vi "random_number.vi"() -> ()   [LabVIEW 2018]
panel:
  out "波形图":dbl[](graph)
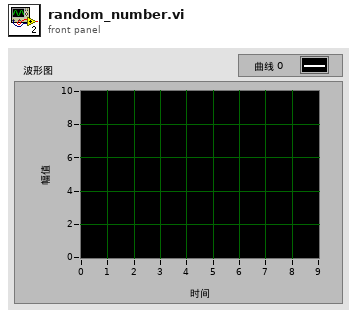
[diagram p1: front panel]
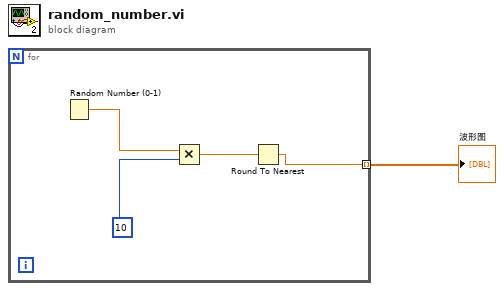
[diagram p0: block diagram]
diagram:
  n1 = for {
    tunnel: [w2] -> w1 mode=indexing
    n2 = Random Number (0-1)() -> (number: 0 to 1=w5:dbl)
    n3 = Multiply(x=w5, y=10) -> (x*y=w3:dbl)
    n4 = Round To Nearest(number=w3) -> (nearest integer value=w2:dbl)
  }
  "波形图" <- w1
